vi "Decode Words to Parameters.vi"(8 "error in":errorcluster, 9 "messages":T1[](array[typedef]), 10 "data words":u16[](array[numeric])=array[4097 elements] format="%04x", 11 "message index":i32) -> (0 "error out":errorcluster, 3 "Values":dbl[](array[numeric]))   [LabVIEW 2020, in "Ballard MIL-STD-1553 Engine.lvlib" / "Implementation.lvlib" / "Rx Execution Unit.lvclass"]
uses:
  Rx Execution Unit.lvclass
  Shared/Message Definition.ctl
  Shared/Message Type.ctl
  Shared/Terminal Endpoint.ctl
  Shared/Address.ctl
  Shared/Parameter Definition.ctl
  e4f9f8f2-2baa-49d9-af10-9a8054fa5784.vi
  81a5383f-fd03-4653-9b89-562a6acab60d.vi
  e4f9f8f2-2baa-49d9-af10-9a8054fa5784.vi/bcb6e6ef-05d7-4341-a691-1e5b866ef5f2.vi
  81a5383f-fd03-4653-9b89-562a6acab60d.vi/0a001d06-2809-4638-8d0b-e017d2157007.vi
  <vilib>/NI/NI VeriStand Encoding and Decoding/BCD Decode Integer.vi
  <vilib>/NI/NI VeriStand Encoding and Decoding/BCD Decode Integer.vi/9a65bfc0-0d77-4ef3-ab58-63df1e1caa90.vi
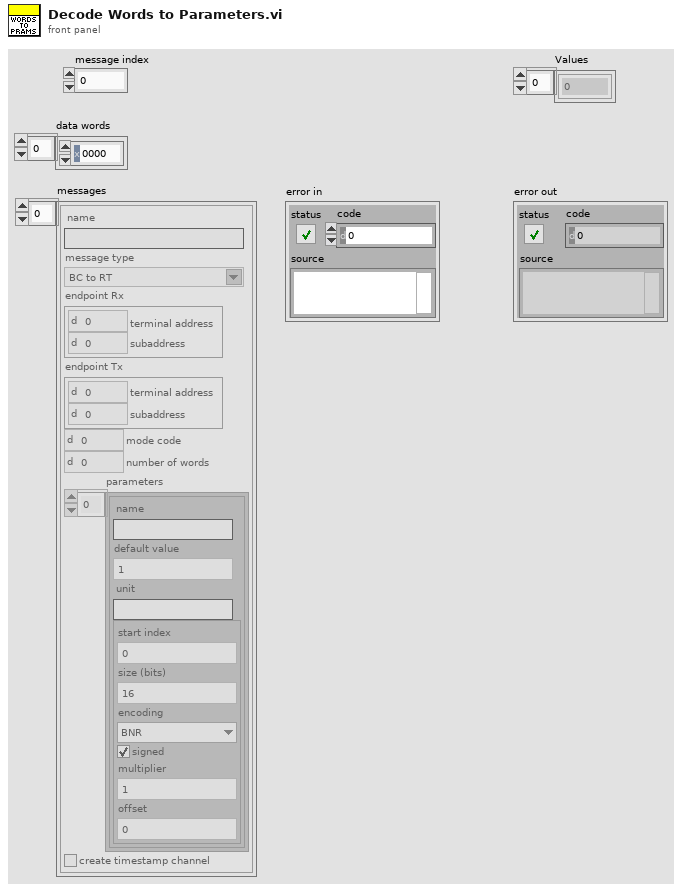
[diagram p1: front panel]
types:
  T1 = typedef "Message Definition.ctl" = cluster{"name":string, "message type":T2, "endpoint Rx":T3, "endpoint Tx":T3, "mode code":u16, "number of words":u16, "parameters":cluster{"name":string, "default value":dbl, "unit":string, "parameter definition":T5}[], "create timestamp channel":bool}
  T2 = typedef "Message Type.ctl" = string
  T3 = typedef "Terminal Endpoint.ctl" = cluster{"terminal address":T4, "subaddress":T4}
  T4 = typedef "Address.ctl" = u16
  T5 = typedef "Parameter Definition.ctl" = cluster{"start index":i32, "size (bits)":i32, "encoding":enum16{"BNR", "BCD", "Discrete"}, "signed":bool, "multiplier":dbl, "offset":dbl}
  T6 = cluster{"name":string, "default value":dbl, "unit":string, "parameter definition":T5}[]
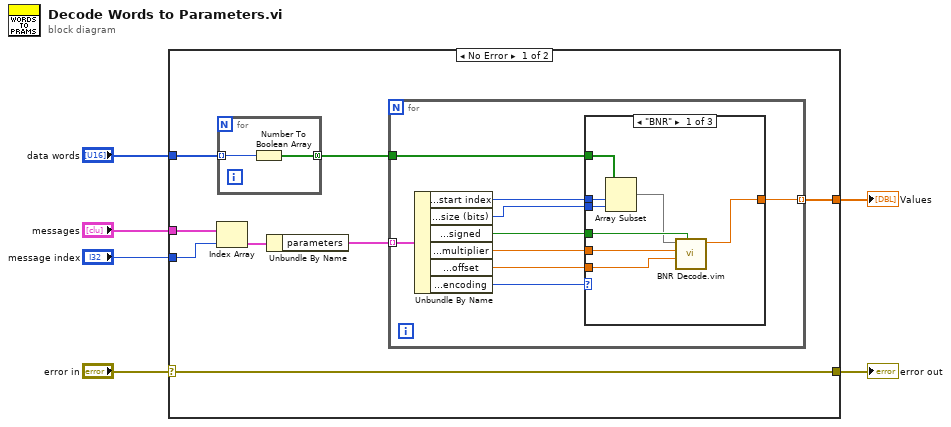
[diagram p0: block diagram]
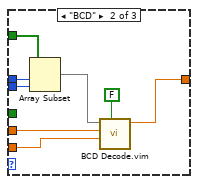
[diagram p2: hidden frame]
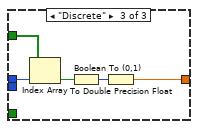
[diagram p3: hidden frame]
diagram:
  n1 = case shown="No Error" "error in" {
    selector: "error in" -> [w14 w47]
    tunnel: [w14 w47] -> w5
    tunnel: "messages" -> [w13 _]
    tunnel: "message index" -> [w12 _]
    tunnel: "data words" -> [w9 _]
    tunnel: [w7 _] -> w1
    frame No Error {
      n2 = Index Array(array=w13, index=w12) -> (element=w11:T1)
      n3 = for {
        tunnel: w9 -> [w16] mode=indexing
        tunnel: [w15] -> w8 mode=concatenating
        n4 = Number To Boolean Array(number=w16) -> (Boolean array=w15:bool[])
      }
      n5 = Unbundle By Name(w11) -> ("parameters"=w10:T6)
      n6 = for {
        tunnel: w10 -> [w25] mode=indexing
        tunnel: w8 -> [w20]
        tunnel: [w17] -> w7 mode=indexing
        n7 = Unbundle By Name(w25) -> ("parameter definition.start index"=w19:i32, "parameter definition.size (bits)"=w18:i32, "parameter definition.signed"=w23:bool, "parameter definition.multiplier"=w22:dbl, "parameter definition.offset"=w21:dbl, "parameter definition.encoding"=w24:enum16{"BNR", "BCD", "Discrete"})
        n8 = case shown="\"BNR\"" w24 {
          tunnel: w23 -> [w29 _ _]
          tunnel: w22 -> [w30 w37 _]
          tunnel: w21 -> [w27 w36 _]
          tunnel: w20 -> [w33 w41 w45]
          tunnel: w19 -> [w32 w40 w46]
          tunnel: w18 -> [w31 w39 _]
          tunnel: [w26 w34 w42] -> w17
          frame "BNR" {
            n9 = Array Subset(array=w33, index=w32, length=w31) -> (w28:bool[])
            n10 = call "BNR Decode.vim"("signed"=w29, "scale offset"=w27, "scale multiplier"=w30, "BNR encoded value"=w28) -> ("value"=w26:dbl)  [unwired: 7 in]
          }
          frame "BCD" {
            n11 = Array Subset(array=w41, index=w40, length=w39) -> (w35:bool[])
            n12 = call "BCD Decode.vim"("signed"=FALSE, "scale offset"=w36, "scale multiplier"=w37, "BCD encoded value"=w35) -> ("value"=w34:dbl)  [unwired: 7 in]
          }
          frame "Discrete" {
            n13 = Index Array(array=w45, index=w46) -> (element=w43:bool)
            n14 = Boolean To (0,1)(Boolean=w43) -> (0, 1=w44:i16)
            n15 = To Double Precision Float(number=w44) -> (double precision float=w42:dbl)
          }
        }
      }
    }
    frame Error {
    }
  }
  "Values" <- w1
  "error out" <- w5
